vi "Do.vi"(8 "error in (no error)":cluster{"状态":bool, "代码":i32, "源":string} caption="错误输入（无错误）", 10 "操作者输入":refnum<class "Actor.lvclass">, 11 "?":refnum<class "Cooler Update Fan Status Msg.lvclass">) -> (0 "error out":cluster{"状态":bool, "代码":i32, "源":string} caption="错误输出", 2 "操作者输出":refnum<class "Actor.lvclass">)   [LabVIEW 2015, in "Evaporative Cooler.lvlib" / "Cooler Update Fan Status Msg.lvclass"]
uses:
  Cooler Update Fan Status Msg.lvclass
  <vilib>/ActorFramework/Actor/Actor.lvclass
  Evaporative Cooler/Evaporative Cooler.lvclass
  Dual Fan/Update Fan Status Msg/Update Fan Status Msg.lvclass/Update Fan Status Msg.ctl
  Dual Fan/Update Fan Status Msg/Update Fan Status Msg.lvclass
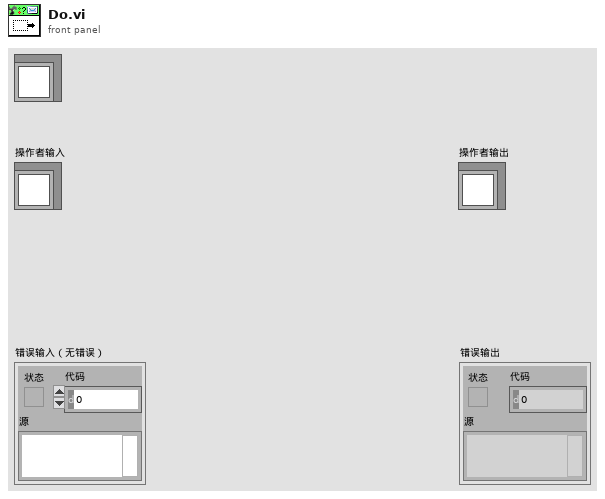
[diagram p1: front panel]
types:
  T1 = typedef "Dual Fan.lvlib/Dual Fan.lvclass/Fan Info.ctl" = cluster{"状态":bool, "故障":bool}
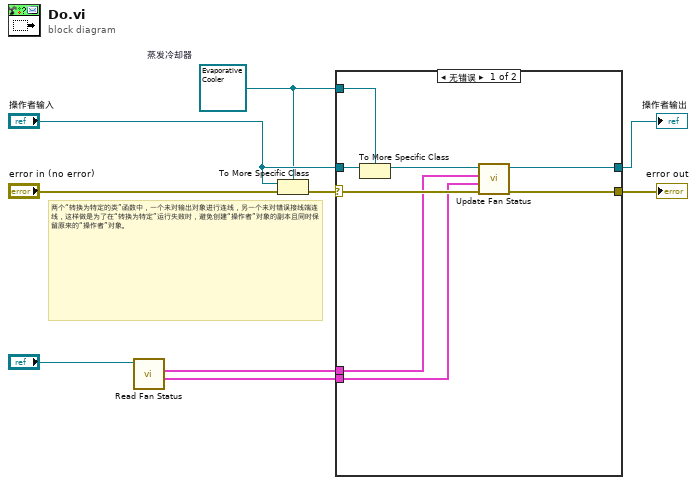
[diagram p0: block diagram]
diagram:
  w4 = refnum<class "Evaporative Cooler.lvclass"> refnum  # 蒸发冷却器
  # "两个“转换为特定的类”函数中，一个未对输出对象进行连线，另一个未对错误接线端连线，这样做是为了在“转换为特定”运行失败时，避免创建“操作者”对象的副本且同时保留原来的“操作者”对象。"
  n1 = call "Read Fan Status.vi"("更新风扇状态消息输入"="?") -> ("风扇B"=w1:T1, "风扇A"=w2:T1)  [unwired: 9 in]
  n2 = To More Specific Class(target class=w4, reference="操作者输入", error in="error in (no error)") -> (error out=w8:errorcluster)  [unwired: 1 out]
  n3 = case shown="无错误" w8 {
    selector: w8 -> [w15 w19]
    tunnel: [w17 w19] -> w7
    tunnel: [w16 w18] -> w6
    tunnel: "操作者输入" -> [w14 w18]
    tunnel: w4 -> [w13 _]
    tunnel: w2 -> [w11 _]
    tunnel: w1 -> [w10 _]
    frame No Error {
      n4 = To More Specific Class(target class=w13, reference=w14) -> (specific class reference=w12:refnum<class "Evaporative Cooler.lvclass">)  [unwired: 1 in, 1 out]
      n5 = call-dynamic "Update Fan Status.vi"("error in (no error)"=w15, "风扇B"=w10, "风扇A"=w11, "蒸发冷却器"=w12) -> ("error out"=w17:cluster{"状态":bool, "代码":i32, "源":string}, "蒸发冷却器"=w16:refnum<class "Evaporative Cooler.lvclass">)  [unwired: 6 in]
    }
    frame Error {
      # "如类型检查失败，则再次将原对象传出。"
    }
  }
  "error out" <- w7
  "操作者输出" <- w6
